vi "RS.vi"(2 "R":bool, 3 "S":bool) -> (0 "~Q":bool=TRUE, 1 "Q":bool)   [LabVIEW 2019, in "Triggers.lvlib"]
uses:
  Triggers.lvlib
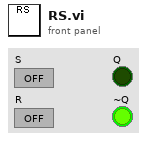
[diagram p1: front panel]
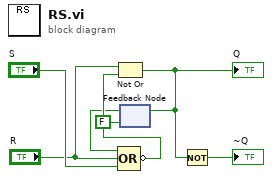
[diagram p0: block diagram]
diagram:
  n1 = feedback #1(FALSE) -> (w5:bool)
  n2 = Compound Arithmetic op=OR(w5, "R", "S") -> (invert w7:bool)
  n3 = Not Or(1:w7, 2:"R") -> (0:w4:bool)
  "Q" <- w4
  n4 = feedback-in #1(w4) -> ()
  n5 = Not(x=w4) -> (.not. x?=→"~Q":bool)
